vi "Read Element of Log_OccupancyGrid.vi"(8 "error in (no error)":errorcluster, 10 "indices":i32[](array[numeric]), 11 "Probabilistic_OccupancyGrid in":refnum<class "Probabilistic_OccupancyGrid.lvclass">) -> (0 "error out":errorcluster, 2 "Numeric":dbl, 3 "Probabilistic_OccupancyGrid out":refnum<class "Probabilistic_OccupancyGrid.lvclass">)   [LabVIEW 2017, in "Probabilistic_OccupancyGrid.lvclass"]
uses:
  Probabilistic_OccupancyGrid.lvclass
  Probabilistic_OccupancyGrid.lvclass/Probabilistic_OccupancyGrid.ctl
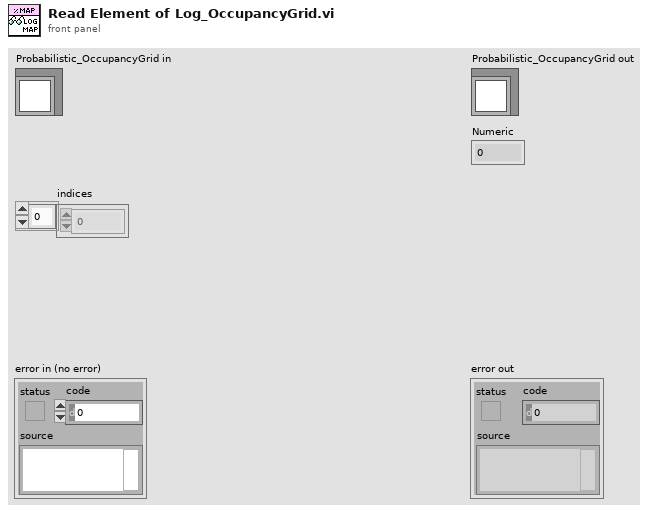
[diagram p1: front panel]
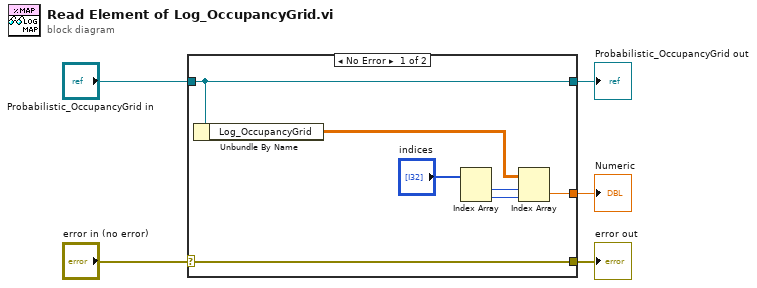
[diagram p0: block diagram]
diagram:
  n1 = case shown="No Error" "error in (no error)" {
    selector: "error in (no error)" -> [w12 w13]
    tunnel: [w12 w13] -> w4
    tunnel: [w11 w14] -> w2
    tunnel: "Probabilistic_OccupancyGrid in" -> [w11 w14]
    tunnel: [w10 _] -> w1
    frame No Error {
      n2 = Unbundle By Name(w11) -> ("Log_OccupancyGrid"=w6:dbl[][])
      n3 = Index Array(array="indices") -> (element #1=w8:i32, element #2=w7:i32)  [unwired: 2 in]
      n4 = Index Array(array=w6, index (row)=w8, index (col)=w7) -> (element=w10:dbl)
    }
    frame Error {
    }
  }
  "error out" <- w4
  "Probabilistic_OccupancyGrid out" <- w2
  "Numeric" <- w1
